vi "SalvaImpostazioni_INPUT.vi"(11 "Array Misure Input":dbl[](array[numeric])) -> ()   [LabVIEW 2016]
uses:
  TypeDef/ClusterCaratteristicheMisura_INPUT.ctl
panel:
  in  "Cluster Caratteriestiche Misura":T1
  in  "Stop":bool
  in  "Carica Impostazioni":bool
  out "Numero di misure":i32
  in  "Salva Impostazioni":bool
  in  "Array ClusterCaratteristicheMisura":T1[](array[typedef])
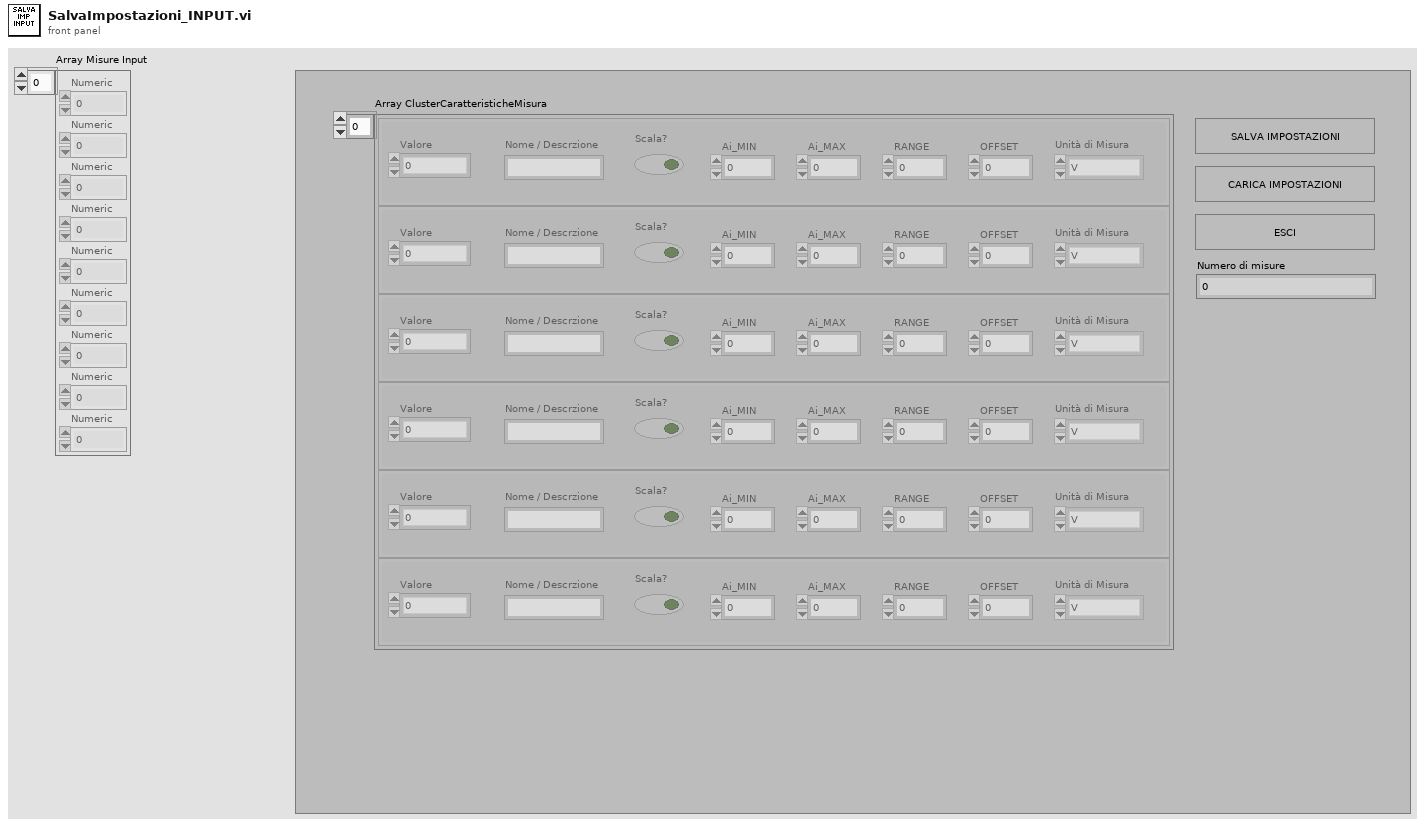
[diagram p1: front panel]
types:
  T1 = typedef "ClusterCaratteristicheMisura_INPUT.ctl" = cluster{"Nome / Descrzione":string, "Scala?":bool, "Ai_MIN":dbl, "Ai_MAX":dbl, "RANGE":dbl, "OFFSET":dbl, "Unità di Misura":T2, "Valore":dbl}
  T2 = typedef "UnitàMisura.ctl" = enum16{"V", "mA", "Bar", "RPM", "m3/s", "m3/min", "m3/h", "l/s", "l/min", "in3/min", "ft3/min", "gpm", "igpm", "igph"}
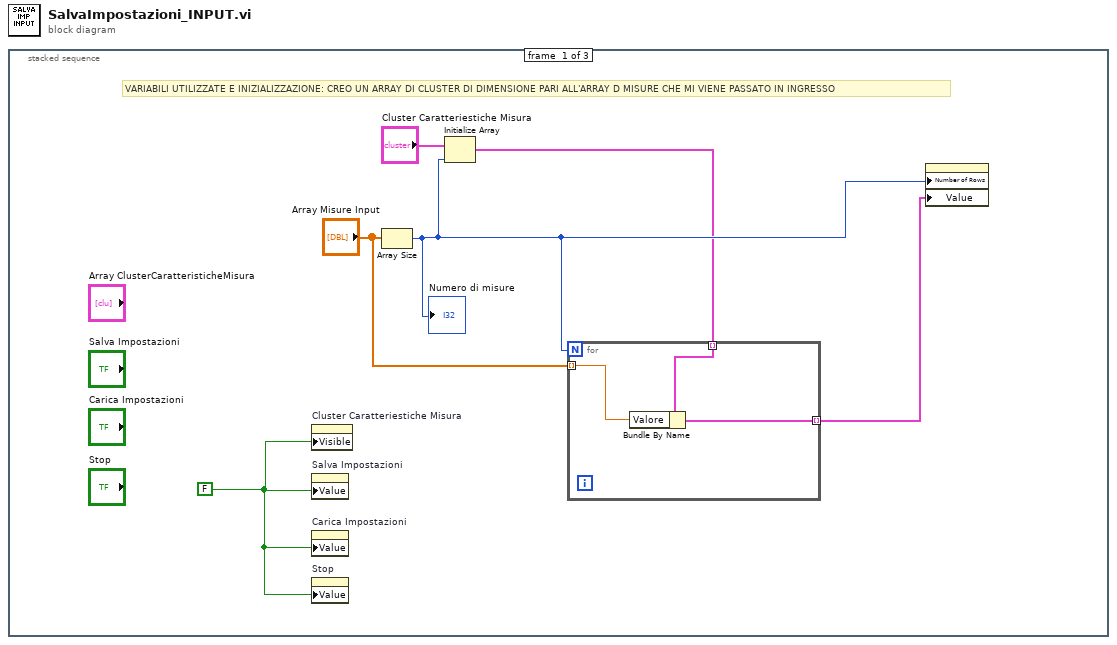
[diagram p0: block diagram]
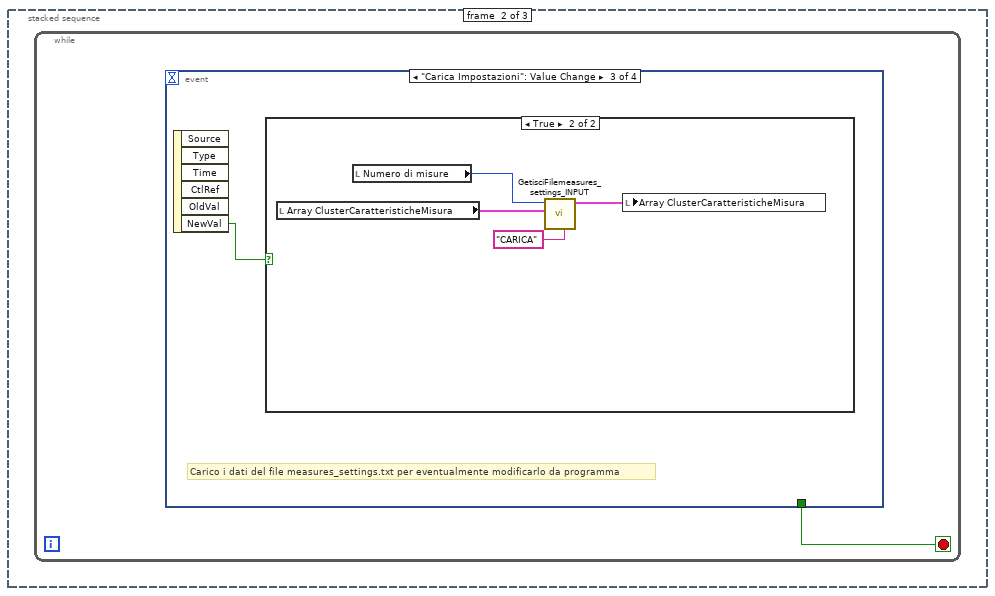
[diagram p2: hidden frame]
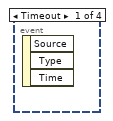
[diagram p3: hidden frame]
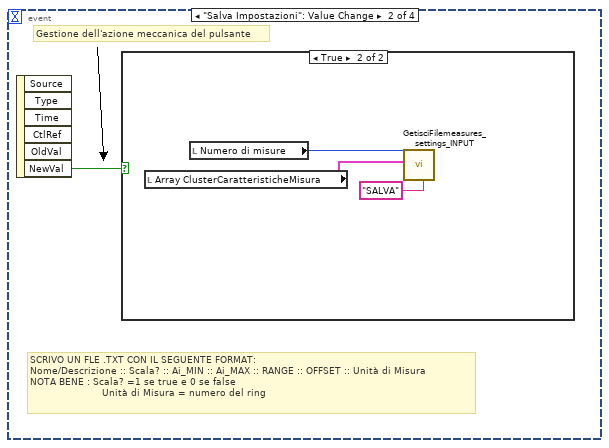
[diagram p4: hidden frame]
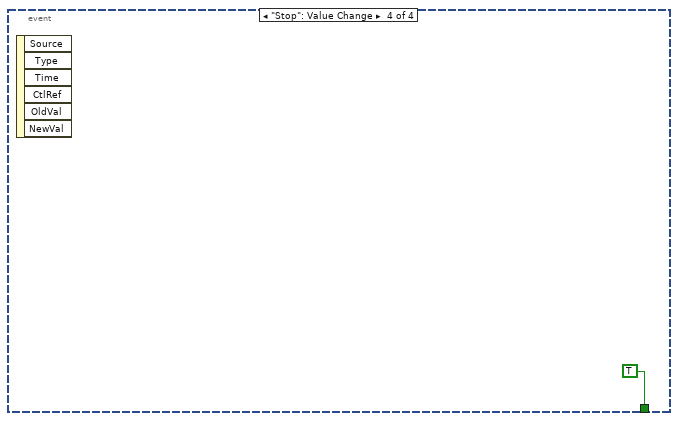
[diagram p7: hidden frame]
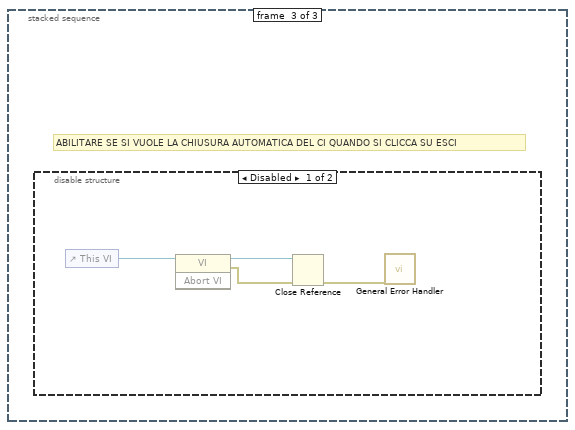
[diagram p8: hidden frame]
diagram:
  n1 = stacked-sequence {
    frame #0 {
      w1 = FALSE ("Salva Impostazioni")
      # "VARIABILI UTILIZZATE E INIZIALIZZAZIONE: CREO UN ARRAY DI CLUSTER DI DIMENSIONE PARI ALL'ARRAY D MISURE CHE MI VIENE PASSATO IN INGRESSO"
      n2 = property on="Cluster Caratteriestiche Misura" class="Clust (strict)"("Visible"=w1) -> ()  [unwired: 2 in, 2 out]
      n3 = property on="Salva Impostazioni" class="Bool (strict)"("Value"=w1) -> ()  [unwired: 2 in, 2 out]
      n4 = property on="Carica Impostazioni" class="Bool (strict)"("Value"=w1) -> ()  [unwired: 2 in, 2 out]
      n5 = property on="Stop" class="Bool (strict)"("Value"=w1) -> ()  [unwired: 2 in, 2 out]
      n6 = Array Size(array="Array Misure Input") -> (size(s)=w4:i32)
      "Numero di misure" <- w4
      n7 = Initialize Array("Cluster Caratteriestiche Misura", w4) -> (w3:T1[])
      n8 = for {
        N: w4 -> [_]
        tunnel: "Array Misure Input" -> [w9] mode=indexing
        tunnel: w3 -> [w8] mode=indexing
        tunnel: [w7] -> w2 mode=indexing
        n9 = Bundle By Name(cluster=w8, "Valore"=w9) -> (w7:T1)
      }
      n10 = property on="Array ClusterCaratteristicheMisura" class="Arr (strict)"("Number of Rows"=w4, "Value"=w2) -> ()  [unwired: 2 in, 2 out]
    }
    frame #1 {
      n11 = while {
        stop <- w10 stop-if-true
        n12 = event shown="[2] \"Carica Impostazioni\": Value Change" {
          selector: _ -> [_ _ _ _]
          dyn-events: _ -> [_ _ _ _]
          timeout: _ -> [_ _ _ _]
          tunnel: [_ _ _ TRUE] -> w10
          event Timeout {
            n13 = event-data() -> ()  [unwired: 1 in, 3 out]
          }
          event "Salva Impostazioni": Value Change {
            # "Gestione dell'azione meccanica del pulsante"
            # "SCRIVO UN FLE .TXT CON IL SEGUENTE FORMAT:\nNome/Descrizione :: Scala? :: Ai_MIN :: Ai_MAX :: RANGE :: OFFSET :: Unità di Misura \nNOTA BENE : Scala? =1 se true e 0 se false\n                        Unità di Misura = numero del ring"
            n14 = event-data() -> ("NewVal"=w11:bool)  [unwired: 1 in, 5 out]
            n15 = case shown="True" w11 {
              frame False {
              }
              frame True {
                n16 = local read "Array ClusterCaratteristicheMisura"() -> (w13:T1[])
                n17 = local read "Numero di misure"() -> (w14:i32)
                n18 = call "GetisciFilemeasures_settings_INPUT.vi"("Numero Misure"=w14, "Array ClusterCaratteristicheMisura IN"=w13, "Azione"="SALVA") -> ()  [unwired: 7 in, 1 out]
              }
            }
          }
          event "Carica Impostazioni": Value Change {
            # "Carico i dati del file measures_settings.txt per eventualmente modificarlo da programma"
            n19 = event-data() -> ("NewVal"=w15:bool)  [unwired: 1 in, 5 out]
            n20 = case shown="True" w15 {
              frame False {
              }
              frame True {
                n21 = local read "Array ClusterCaratteristicheMisura"() -> (w18:T1[])
                n22 = local read "Numero di misure"() -> (w17:i32)
                n23 = call "GetisciFilemeasures_settings_INPUT.vi"("Numero Misure"=w17, "Array ClusterCaratteristicheMisura IN"=w18, "Azione"="CARICA") -> ("Array ClusterCaratteristicheMisura OUT"=w16:T1[])  [unwired: 7 in]
                n24 = local write "Array ClusterCaratteristicheMisura"(w16) -> ()
              }
            }
          }
          event "Stop": Value Change {
            n25 = event-data() -> ()  [unwired: 1 in, 6 out]
          }
        }
      }
    }
    frame #2 {
      # "ABILITARE SE SI VUOLE LA CHIUSURA AUTOMATICA DEL CI QUANDO SI CLICCA SU ESCI"
      n26 = disable-structure shown="Disabled" {
        frame Disabled {
          n27 = control-ref of="This VI"() -> (w24:refnum<vi>)
          n28 = invoke class="VI" method="Abort VI"(reference=w24) -> (reference out=w23:refnum<vi>, error out=w21:errorcluster)  [unwired: 2 in, 1 out]
          n29 = Close Reference(reference=w23, error in (no error)=w21) -> (error out=w22:errorcluster)
          n30 = call <vilib>:"General Error Handler.vi"("error in (no error)"=w22) -> ()  [unwired: 10 in, 5 out]
        }
        frame Enabled {
        }
      }
    }
  }
